vi "NI5112.set bin width.vi"(0 "i ref in":refnum<vi>, 2 "bin width [us]":dbl format="%.2f", 3 "ms timeout (100)":i32=100, 5 "error in (no error)":errorcluster) -> (14 "i ref out":refnum<vi>, 17 "timed out":bool, 19 "error out":errorcluster)   [LabVIEW 2014, in "NI5112.lvlib"]
uses:
  NI5112.lvlib
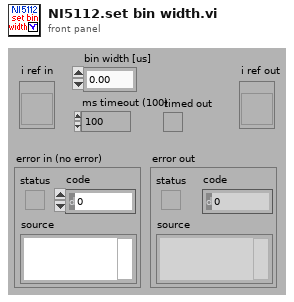
[diagram p1: front panel]
types:
  T1 = typedef "NI5112.lvlib/NI5112.i attribute.ctl" = cluster{"HWChannel":string, "instrument handle":refnum<k15>, "BinWidth":dbl, "vertical offset":dbl, "vertical range":dbl, "DataBPR":i32, "5112BPR":i32, "FullSpeed":bool, "discrLevel":dbl, "DoDiscr":bool, "VerCoupling":string}
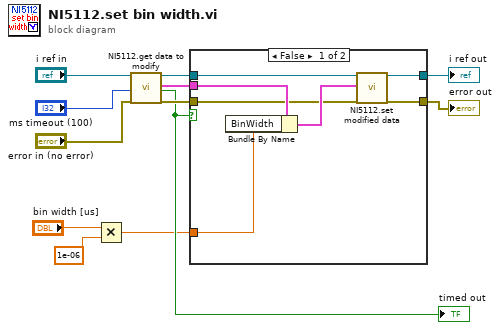
[diagram p0: block diagram]
diagram:
  n1 = Multiply(x="bin width [us]", y=1e-06) -> (x*y=w1:dbl)
  n2 = call "NI5112.get data to modify.vi"("i ref in"="i ref in", "ms timeout (10000)"="ms timeout (100)", "error in (no error)"="error in (no error)") -> ("i ref out"=w8:refnum<vi>, "i attribute"=w6:T1, "timed out"=w4:bool, "error out"=w7:errorcluster)  [unwired: 13 in]
  "timed out" <- w4
  n3 = case shown="False" w4 {
    tunnel: [w19 w20] -> w10
    tunnel: [w18 w21] -> w9
    tunnel: w8 -> [w17 w21]
    tunnel: w7 -> [w13 w20]
    tunnel: w6 -> [w16 _]
    tunnel: w1 -> [w14 _]
    frame False {
      n4 = Bundle By Name(cluster=w16, "BinWidth"=w14) -> (w15:T1)
      n5 = call "NI5112.set modified data.vi"("i ref in"=w17, "i attribute"=w15, "error in (no error)"=w13) -> ("i ref out"=w18:refnum<vi>, "error out"=w19:errorcluster)  [unwired: 15 in]
    }
    frame True {
    }
  }
  "error out" <- w10
  "i ref out" <- w9
